vi "ApplyLayoutToObject.vi"(5 "scaling settings":T1={"scaling factor"={"horizontal"=1.0, "vertical"=1.0}, "scaling to ignore"=variant} {"scaling factor"."vertical" min=0.0; "scaling factor"."horizontal" min=0.0}, 7 "properties to ignore":variant, 8 "error in (no error)":errorcluster, 10 "GObj Refnum":refnum<vi>, 11 "Object Layout in":refnum<class "Pane Layout.lvclass">) -> (0 "error out":errorcluster, 3 "Object Layout out":refnum<class "Pane Layout.lvclass">)   [LabVIEW 2010, in "NI_SE_Front Panel Layout.lvlib" / "Pane Layout.lvclass"]
doc: "Apply layout information to the GObj Refnum."
uses:
  Pane Layout.lvclass
  Scaling Factor_Options.ctl
  XY Scaling Factor.ctl
  Object Layout/Object Layout.lvclass
  Pane Layout.lvclass/Pane Layout.ctl
  Properties To Ignore.vi
  NI_SE_Front Panel Layout.lvlib
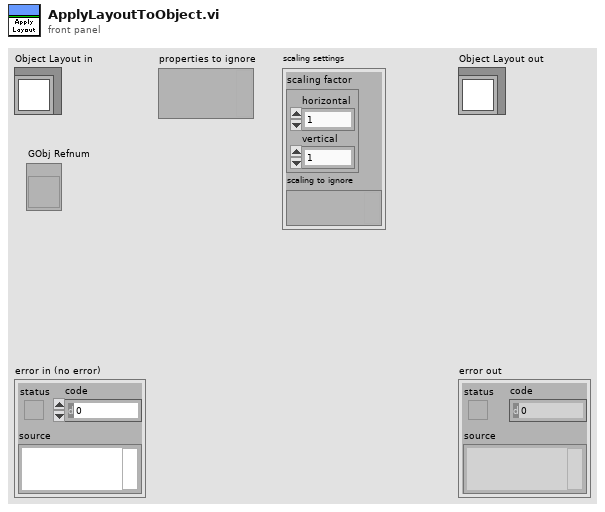
[diagram p1: front panel]
types:
  T1 = typedef "NI_SE_Front Panel Layout.lvlib/Scaling Factor_Options.ctl" = cluster{"scaling factor":T2, "scaling to ignore":variant}
  T2 = typedef "NI_SE_Front Panel Layout.lvlib/XY Scaling Factor.ctl" = cluster{"horizontal":dbl, "vertical":dbl}
  T3 = typedef "LVPointTypeDef.ctl" = cluster{"Horizontal":i16, "Vertical":i16}
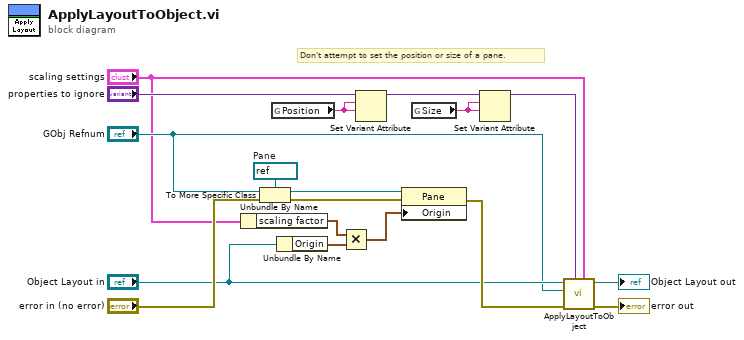
[diagram p0: block diagram]
diagram:
  w8 = refnum<vi> refnum  # Pane
  # "Don't attempt to set the position or size of a pane."
  n1 = Unbundle By Name("scaling settings") -> ("scaling factor"=w3:T2)
  n2 = To More Specific Class(target class=w8, reference="GObj Refnum", error in="error in (no error)") -> (specific class reference=w7:refnum<vi>, error out=w4:errorcluster)
  n3 = global read "Properties To Ignore.vi" "Position"() -> (w2:string)
  n4 = Unbundle By Name("Object Layout in") -> ("Origin"=w6:T3)
  n5 = Multiply(x=w3, y=w6) -> (x*y=w5:T2)
  n6 = Set Variant Attribute(Variant="properties to ignore", name=w2, value=w2) -> (Variant out=w10:variant)  [unwired: 1 in, 2 out]
  n7 = property class="Pane"(reference=w7, error in=w4, "Origin"=w5) -> (error out=w14:errorcluster)  [unwired: 1 out]
  n8 = global read "Properties To Ignore.vi" "Size"() -> (w1:string)
  n9 = Set Variant Attribute(Variant=w10, name=w1, value=w1) -> (Variant out=w9:variant)  [unwired: 1 in, 2 out]
  n10 = call-parent "ApplyLayoutToObject.vi"("scaling settings"="scaling settings", "properties to ignore"=w9, "error in (no error)"=w14, "GObj Refnum"="GObj Refnum", "Object Layout in"="Object Layout in") -> ("error out"=→"error out":errorcluster, "Object Layout out"=→"Object Layout out":refnum<class "Pane Layout.lvclass">)  [unwired: 5 in]
